vi "Write #Frames.vi"(8 "error in (no error)":errorcluster, 10 "#Frames":u32, 11 "Start ExperimentSet Msg in":refnum<class "Start ExperimentSet Msg.lvclass">) -> (0 "error out":errorcluster, 3 "Start ExperimentSet Msg out":refnum<class "Start ExperimentSet Msg.lvclass">)   [LabVIEW 2014]
uses:
  Start ExperimentSet Msg.lvclass
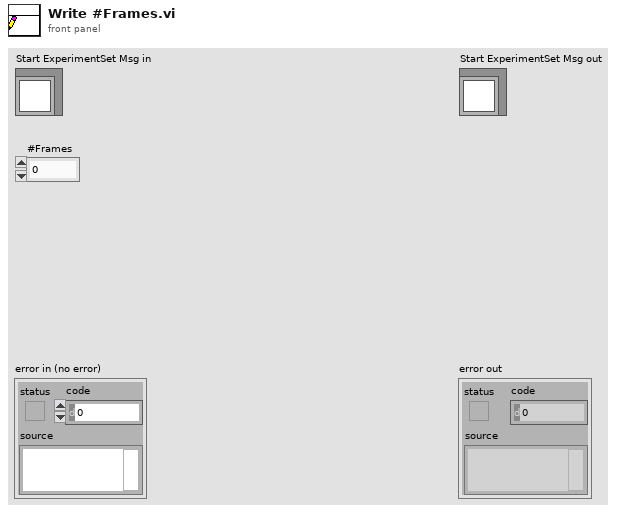
[diagram p1: front panel]
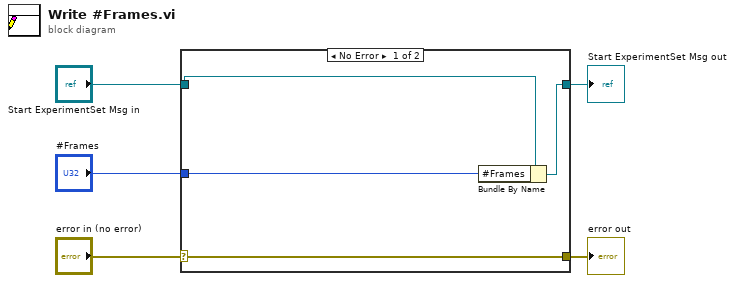
[diagram p0: block diagram]
diagram:
  n1 = case shown="No Error" "error in (no error)" {
    selector: "error in (no error)" -> [w9 w10]
    tunnel: [w9 w10] -> w4
    tunnel: [w7 w11] -> w2
    tunnel: "Start ExperimentSet Msg in" -> [w8 w11]
    tunnel: "#Frames" -> [w6 _]
    frame No Error {
      n2 = Bundle By Name(cluster=w8, "#Frames"=w6) -> (w7:refnum<class "Start ExperimentSet Msg.lvclass">)
    }
    frame Error {
    }
  }
  "error out" <- w4
  "Start ExperimentSet Msg out" <- w2
